vi "ni5660 Configure Reference Clock.vi"(0 "receiver info in":T1, 5 "clock source":string(combo)="On Board Clock", 7 "drive backplane clock":enum16{"FALSE", "TRUE"}(ring), 9 "digitizer PLL lock time (sec)":dbl=1.0, 11 "error in (no error)":errorcluster) -> (4 "receiver info out":T1, 15 "error out":errorcluster)   [LabVIEW 2011]
doc: "Use this function to configure the reference clock source for the RF Signal Analyzer. Reference clock source options include the high-stability oven-controlled crystal oscillator (OCXO) onboard the RF downconverter module (On Board Clock), a 10 MHz reference clock from an external source (Ref In), or the PXI backplane (PXI Clock 10). You can optionally use this VI to drive the PXI backplane using the specified reference clock source."
uses:
  <vilib>/addons/Modulation/niScope/controls/mod_Modulation Settings.ctl
  Instance           7 40Saved   ni5660 Configure Reference Clock .vi
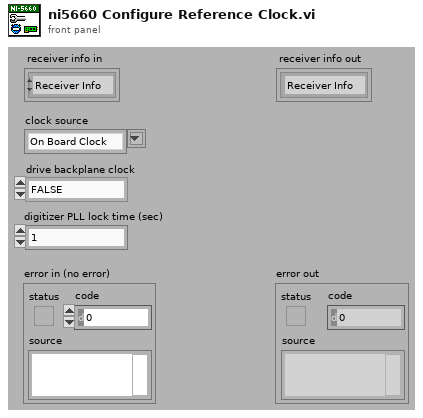
[diagram p1: front panel]
types:
  T1 = typedef "mod_Modulation Settings.ctl" = cluster{enum16{"Receiver Info"}, variant}
  T2 = enum32{"Drive 10 MHz PXI Backplane Clock", "Internal", "Lock To 10 MHz PXI Backplane Clock", "External", "Drive 10 MHz PXI Backplane Clock External"}
  T3 = typedef "mod_Readable Attributes Cluster.ctl" = cluster{"carrier":cluster{"frequency":dbl}, "receiver":cluster{"handles":cluster{"niTuner taskID":i32, "niScope handle":refnum<k15>}, "RFSA":cluster{"reference level":i32, "RF attenuation":i32}, "data format":enum16{"real", "complex modulated (array)", "complex modulated (interleaved)"}, "auto suppress SW IQ":enum16{"off", "on"}, "IQ sample rate":dbl, "bandwidth":dbl}}
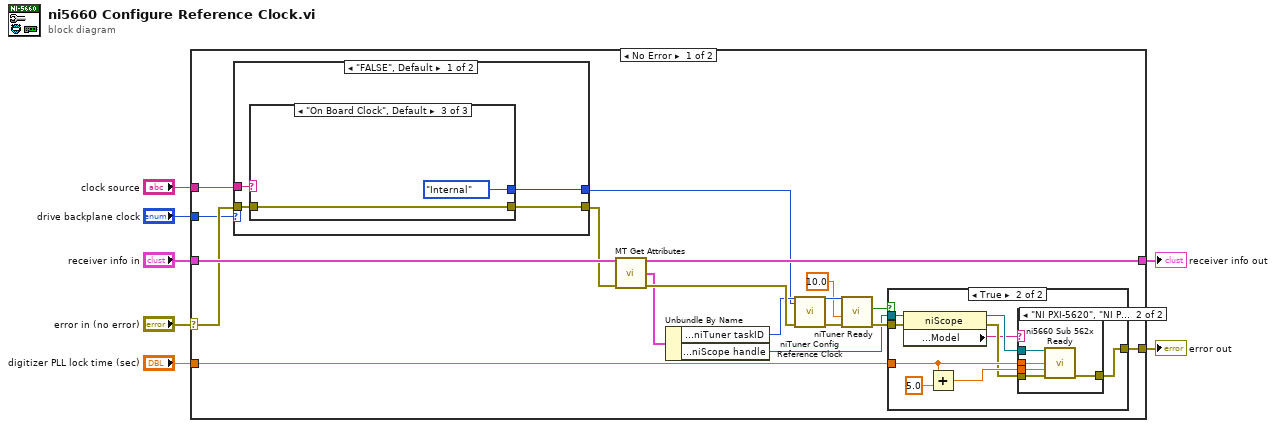
[diagram p0: block diagram]
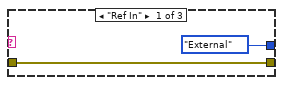
[diagram p2: hidden frame]
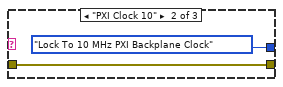
[diagram p3: hidden frame]
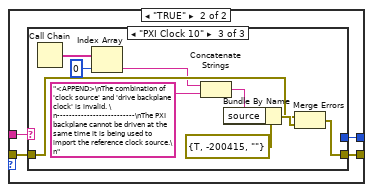
[diagram p4: hidden frame]
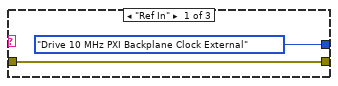
[diagram p5: hidden frame]
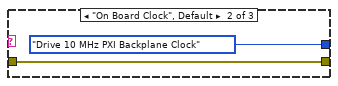
[diagram p6: hidden frame]
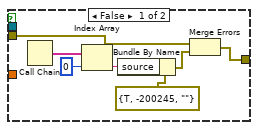
[diagram p7: hidden frame]
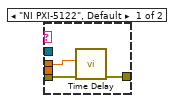
[diagram p8: hidden frame]
diagram:
  n1 = case shown="No Error" "error in (no error)" {
    selector: "error in (no error)" -> [w13 w77]
    tunnel: "receiver info in" -> [w25 w78]
    tunnel: [w19 w78] -> w6
    tunnel: [w18 w77] -> w4
    tunnel: "digitizer PLL lock time (sec)" -> [w16 _]
    tunnel: "drive backplane clock" -> [w11 _]
    tunnel: "clock source" -> [w14 _]
    frame No Error {
      n2 = case shown="\"FALSE\", Default" w11 {
        tunnel: w14 -> [w29 w38]
        tunnel: [w28 w39] -> w15
        tunnel: w13 -> [w27 w37]
        tunnel: [w26 w36] -> w12
        frame "FALSE", Default {
          n3 = case shown="\"On Board Clock\", Default" w29 {
            tunnel: [T2."External" ("reference configuration") T2."Lock To 10 MHz PXI Backplane Clock" ("reference configuration") T2."Internal" ("reference configuration")] -> w28
            tunnel: w27 -> [w30 w32 w34]
            tunnel: [w30 w32 w34] -> w26
            frame "Ref In" {
            }
            frame "PXI Clock 10" {
            }
            frame "On Board Clock", Default {
            }
          }
        }
        frame "TRUE" {
          n4 = case shown="\"PXI Clock 10\"" w38 {
            tunnel: [T2."Drive 10 MHz PXI Backplane Clock External" ("reference configuration") T2."Drive 10 MHz PXI Backplane Clock" ("reference configuration") _] -> w39
            tunnel: w37 -> [w40 w42 w48]
            tunnel: [w40 w42 w47] -> w36
            frame "Ref In" {
            }
            frame "On Board Clock", Default {
            }
            frame "PXI Clock 10" {
              n5 = Call Chain() -> (call chain=w52:string[])
              n6 = Index Array(array=w52, index=0) -> (element=w46:string)
              n7 = Concatenate Strings(w46, "<APPEND>\nThe combination of 'clock source' and 'drive backplane clock' is invalid. \n--------------------------\nThe PXI backplane cannot be driven at the same time it is being used to import the reference clock source.\n") -> (w45:string)
              n8 = Bundle By Name(cluster=errorcluster {"status"=TRUE, "code"=-200415, "source"=""} ("error out"), "source"=w45) -> (w49:errorcluster)
              n9 = Merge Errors(w48, w49) -> (w47:errorcluster)
            }
          }
        }
      }
      n10 = call <vilib>:"MT Get Attributes.vi"("receiver info in"=w25, "error in (no error)"=w12) -> ("receiver info out"=w19:T1, "attributes"=w20:T3, "error out"=w24:errorcluster)  [unwired: 11 in]
      n11 = Unbundle By Name(w20) -> ("receiver.handles.niTuner taskID"=w23:i32, "receiver.handles.niScope handle"=w8:refnum<k15>)
      n12 = call <instrlib>:"niTuner Config Reference Clock.vi"("error in"=w24, "reference configuration"=w15, "taskID in"=w23) -> ("error out"=w22:errorcluster, "taskID out"=w21:i32)  [unwired: 6 in]
      n13 = call <instrlib>:"niTuner Ready.vi"("error in"=w22, "timeout"=10.0, "taskID in"=w21) -> ("error out"=w9:errorcluster, "ready"=w10:bool)  [unwired: 6 in, 1 out]
      n14 = case shown="True" w10 {
        tunnel: w9 -> [w59 w64]
        tunnel: [w56 w68] -> w18
        tunnel: w16 -> [_ w66]
        tunnel: w8 -> [_ w62]
        frame False {
          n15 = Call Chain() -> (call chain=w55:string[])
          n16 = Index Array(array=w55, index=0) -> (element=w53:string)
          n17 = Bundle By Name(cluster=errorcluster {"status"=TRUE, "code"=-200245, "source"=""} ("error out"), "source"=w53) -> (w57:errorcluster)
          n18 = Merge Errors(w59, w57) -> (w56:errorcluster)
        }
        frame True {
          n19 = property class="niScope"(reference=w62, error in=w64) -> (reference out=w61:refnum<k15>, error out=w63:errorcluster, "Inherent IVI Attributes:Instrument Identification:Model"=w60:string)
          n20 = Add(x=w66, y=5.0 ("max timeout (sec)")) -> (x+y=w65:dbl)
          n21 = case shown="\"NI PXI-5620\", \"NI PXI-5621\"" w60 {
            tunnel: w63 -> [w71 w76]
            tunnel: [w70 w75] -> w68
            tunnel: w66 -> [w69 w74]
            tunnel: w65 -> [_ w73]
            tunnel: w61 -> [_ w72]
            frame "NI PXI-5122", Default {
              n22 = call "Time Delay"("error in (no error)"=w71, "Delay Time (s)"=w69) -> ("error out"=w70:errorcluster)  [unwired: 9 in]
            }
            frame "NI PXI-5620", "NI PXI-5621" {
              n23 = call <instrlib>:"ni5660 Sub 562x Ready.vi"("instrument handle in"=w72, "PLL lock time (sec)"=w74, "max timeout (sec)"=w73, "error in (no error)"=w76) -> ("error out"=w75:errorcluster)  [unwired: 10 in, 1 out]
            }
          }
        }
      }
    }
    frame Error {
    }
  }
  "error out" <- w4
  "receiver info out" <- w6
